vi "Init Runtime.vi"(8 "error in (no error)":errorcluster, 11 "OnTheFlyReport Config in":refnum<class "OnTheFlyReport Config.lvclass">) -> (0 "error out":errorcluster, 2 "Report.lvclass":refnum<class "Report.lvclass">, 3 "OnTheFlyReport Config out":refnum<class "OnTheFlyReport Config.lvclass">)   [LabVIEW 2015, in "OnTheFlyReport Config.lvclass"]
doc: "This VI returns a runtime class for the Report using the configuration provided."
uses:
  OnTheFlyReport Config.lvclass
  Generic/Execution/Report.lvclass
  Execution/OnTheFlyReport.lvclass
  OnTheFlyReport Config.lvclass/OnTheFlyReport Config.ctl
  Report Formatters/Base Class/Config/Formatter Config.lvclass
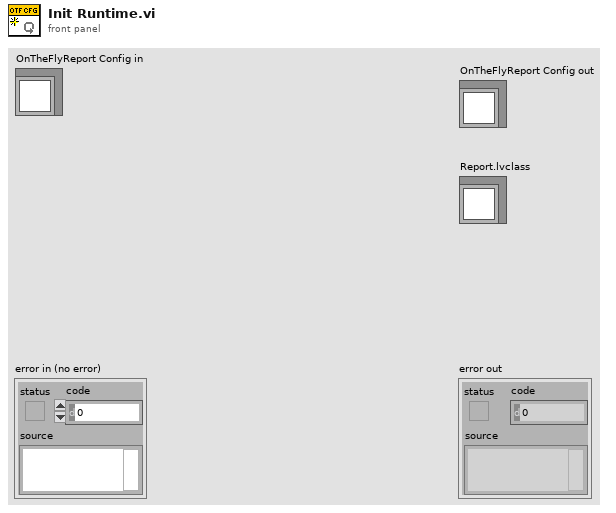
[diagram p1: front panel]
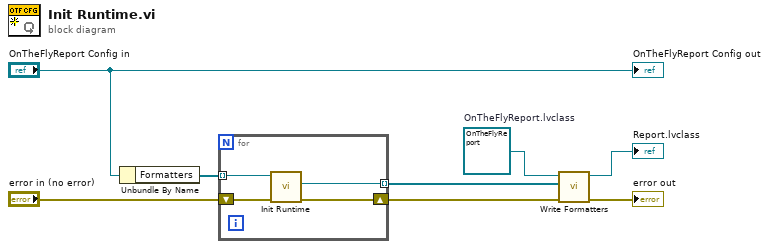
[diagram p0: block diagram]
diagram:
  w7 = refnum<class "OnTheFlyReport.lvclass"> refnum  # OnTheFlyReport.lvclass
  n1 = Unbundle By Name("OnTheFlyReport Config in") -> ("Formatters"=w5:refnum<class "Formatter Config.lvclass">[])
  n2 = for {
    tunnel: w5 -> [w12] mode=indexing
    tunnel: [w11] -> w2 mode=indexing
    shift-right: [w9] -> w3
    shift-left: "error in (no error)" -> [w10]
    n3 = call-dynamic "Init Runtime.vi"("error in (no error)"=w10, "Formatter Config in"=w12) -> ("error out"=w9:errorcluster, "Formatter.lvclass"=w11:refnum<class "Formatter.lvclass">)  [unwired: 7 in, 1 out]
  }
  n4 = call-dynamic "Write Formatters.vi"("error in (no error)"=w3, "Formatters"=w2, "OnTheFlyReport in"=w7) -> ("error out"=→"error out":errorcluster, "OnTheFlyReport out"=→"Report.lvclass":refnum<class "OnTheFlyReport.lvclass">)  [unwired: 7 in]
  "OnTheFlyReport Config out" <- "OnTheFlyReport Config in"
